vi "Transceiver Initialize.vi"(8 "error in (no error)":errorcluster, 11 "Plugin Thread in":refnum<class "Plugin Thread.lvclass">) -> (0 "error out":errorcluster, 3 "Plugin Thread out":refnum<class "Plugin Thread.lvclass">)   [LabVIEW 2017, in "DSF Core.lvlib" / "Plugin Thread.lvclass"]
uses:
  Thread/Plugin/Plugin Thread.lvclass
  Transceiver.lvclass
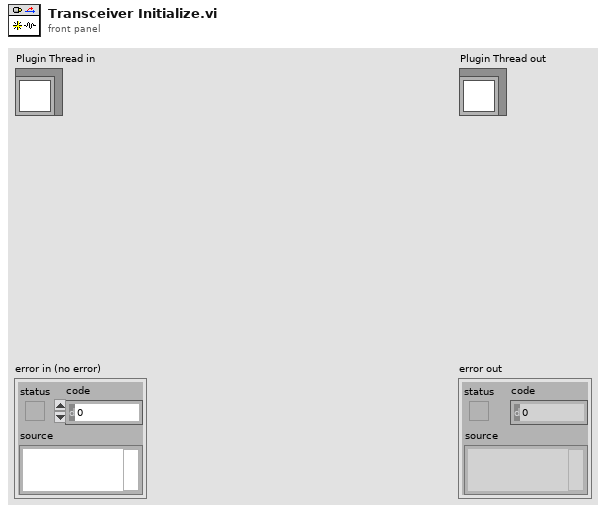
[diagram p1: front panel]
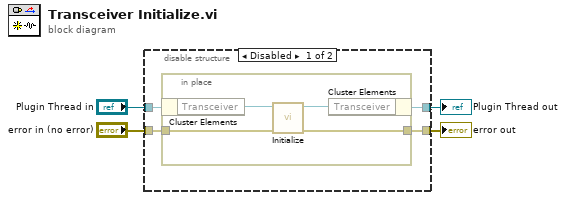
[diagram p0: block diagram]
diagram:
  n1 = disable-structure shown="Disabled" {
    disable-tunnel: [w8 w13] -> w4
    disable-tunnel: "error in (no error)" -> [w7 w13]
    disable-tunnel: "Plugin Thread in" -> [w6 w14]
    disable-tunnel: [w5 w14] -> w1
    frame Disabled {
      n2 = in-place {
        in-place-border: [w12] -> w8
        in-place-border: w7 -> [w11]
        n3 = in-place-cluster #1(w6) -> ("Transceiver"=w10:refnum<class "Transceiver.lvclass">)
        n4 = call-dynamic "Initialize.vi"("error in (no error)"=w11, "Transceiver in"=w10) -> ("error out"=w12:errorcluster, "Transceiver out"=w9:refnum<class "Transceiver.lvclass">)  [unwired: 8 in]
        n5 = in-place-cluster #1("Transceiver"=w9) -> (w5:refnum<class "Plugin Thread.lvclass">)
      }
    }
    frame Enabled {
    }
  }
  "error out" <- w4
  "Plugin Thread out" <- w1
